vi "parse navigation string.vi"(6 "Header":string="T", 8 "Nav String":string="$,G,43,13,230,P,10,20,120,T,10,10,330,L,14,36,110,A,3,5,B,7,8,C,16,20,D,-1,-1,S,08,12,234\r") -> (0 "Valid?":bool, 1 "angle":i32, 2 "y":i32, 3 "x":i32)   [LabVIEW 2013]
doc: "This VI will parse the Tug navigation string for the Tug letters, A for example, and the time, T. It returns a cluster with the Tug / Time and three values as decimals."
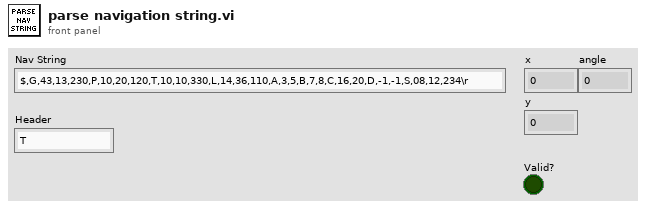
[diagram p1: front panel]
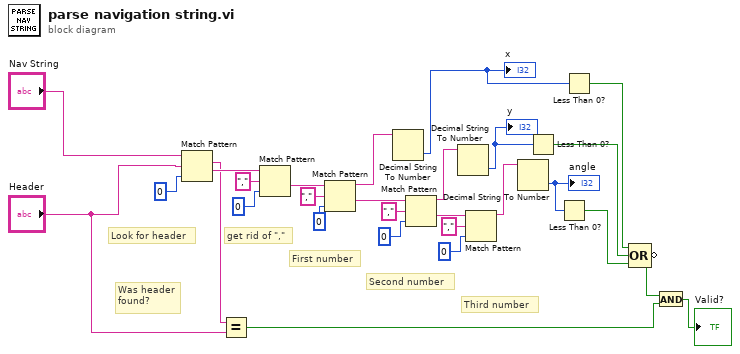
[diagram p0: block diagram]
diagram:
  # "Was header\nfound?"
  # "Third number"
  # "Second number"
  # "First number"
  # "get rid of \",\""
  # "Look for header"
  n1 = Match Pattern(string="Nav String", regular expression="Header", offset (0)=0) -> (match substring=w11:string, after substring=w13:string)  [unwired: 2 out]
  n2 = Equal?(x=w11, y="Header") -> (x = y?=w6:bool)
  n3 = Match Pattern(string=w13, regular expression=",", offset (0)=0) -> (after substring=w14:string)  [unwired: 3 out]
  n4 = Match Pattern(string=w14, regular expression=",", offset (0)=0) -> (before substring=w25:string, after substring=w21:string)  [unwired: 2 out]
  n5 = Decimal String To Number(string=w25) -> (number=w9:i32)  [unwired: 2 in, 1 out]
  "x" <- w9
  n6 = Match Pattern(string=w21, regular expression=",", offset (0)=0) -> (before substring=w22:string, after substring=w17:string)  [unwired: 2 out]
  n7 = Decimal String To Number(string=w22) -> (number=w8:i32)  [unwired: 2 in, 1 out]
  "y" <- w8
  n8 = Match Pattern(string=w17, regular expression=",", offset (0)=0) -> (before substring=w18:string)  [unwired: 3 out]
  n9 = Decimal String To Number(string=w18) -> (number=w7:i32)  [unwired: 2 in, 1 out]
  "angle" <- w7
  n10 = Less Than 0?(x=w8) -> (x < 0?=w4:bool)
  n11 = Less Than 0?(x=w7) -> (x < 0?=w3:bool)
  n12 = Less Than 0?(x=w9) -> (x < 0?=w5:bool)
  n13 = Compound Arithmetic op=OR(w5, w4, w3) -> (invert w2:bool)
  n14 = And(x=w2, y=w6) -> (x .and. y?=→"Valid?":bool)
